vi "Set_Reset_Now.vi"(7 "I2C Channel":u8, 8 "error in (no error)":errorcluster, 11 "LINX Resource In":T1) -> (0 "error out":errorcluster, 3 "LINX Resource Out":T1)   [LabVIEW 2014, in "LMH-LINX.lvlib" / "HMC6352.lvlib"]
uses:
  <vilib>/MakerHub/LINX/Public/Sensors/Orientation/Compass/HMC6352/HMC6352.lvlib
  <vilib>/MakerHub/LINX/Private/Type Defs/LINX Ref.ctl
  <vilib>/MakerHub/LINX/Private/Type Defs/Platform.ctl
  <vilib>/MakerHub/LINX/Private/Type Defs/Interface.ctl
  <vilib>/MakerHub/LINX/Private/Device/Type Defs/LINX Device Config.ctl
  <vilib>/MakerHub/LINX/Private/Device/Type Defs/TCP Config.ctl
  <vilib>/MakerHub/LINX/Private/Device/Type Defs/Channels.ctl
  <vilib>/MakerHub/LINX/Private/Local IO/LinxI2cWrite.vi
  <vilib>/MakerHub/LINX/Public/Utilities/Check Channel.vi
  <vilib>/MakerHub/LINX/Private/Utilties/Generate Error.vi
  <vilib>/MakerHub/LINX/LMH-LINX.lvlib
  <vilib>/MakerHub/LINX/Private/Device/Device.lvlib
panel:
  # "INPUTS"
  # "OUTPUTS"
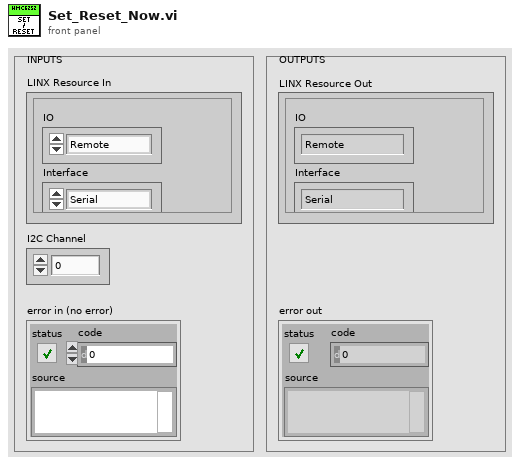
[diagram p1: front panel]
types:
  T1 = typedef "LMH-LINX.lvlib/LINX Ref.ctl" = cluster{"IO":T2, "Interface":T3, "LINX Device Config":T4}
  T2 = typedef "LMH-LINX.lvlib/Platform.ctl" = enum16{"Remote", "Local"}
  T3 = typedef "LMH-LINX.lvlib/Interface.ctl" = enum16{"Serial", "TCP"}
  T4 = typedef "LMH-LINX.lvlib/Device.lvlib/LINX Device Config.ctl" = cluster{"Interface":T3, "COM Port":refnum<visa-resource-name>, "TCP Configuration":T5, "Device Family":u8, "Device ID":u8, "Device Name":string, "TCP Ref":refnum<k5>, "Channels":T6}
  T5 = typedef "LMH-LINX.lvlib/Device.lvlib/TCP Config.ctl" = cluster{"IP Address":string, "Port":u16}
  T6 = typedef "LMH-LINX.lvlib/Channels.ctl" = cluster{"DI":u8[], "DO":u8[], "AI":u8[], "AO":u8[], "PWM":u8[], "QE":u8[], "UART":u8[], "I2C 2":u8[], "SPI":u8[], "CAN":u8[], "Servo":u8[], "AI Ref (V)":dbl, "AI Resolution (Bits)":u8, "AO Ref (V)":dbl, "AO Resolution (Bits)":u8}
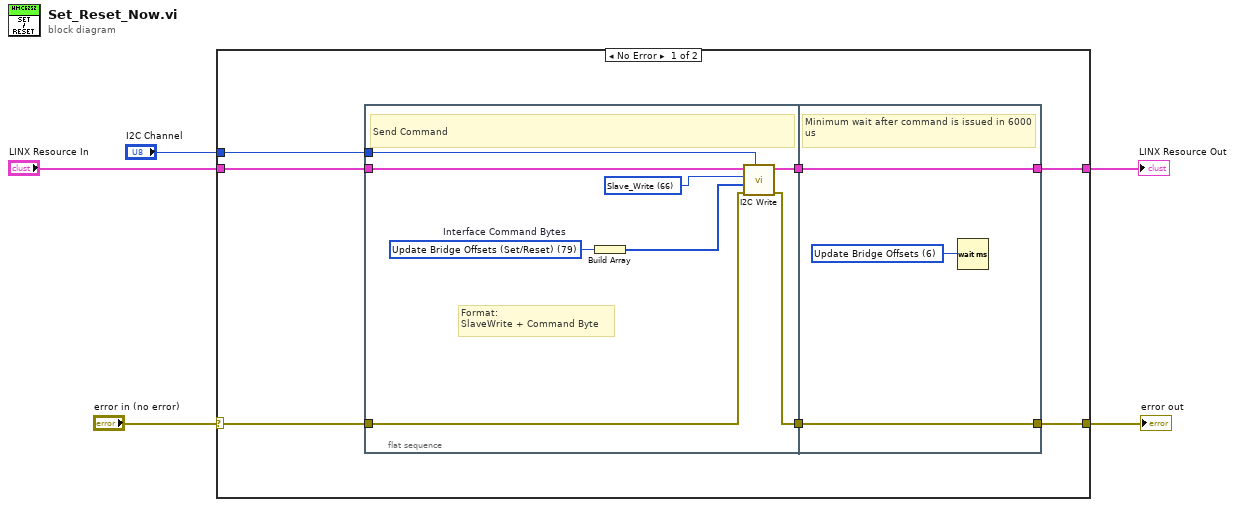
[diagram p0: block diagram]
diagram:
  n1 = case shown="No Error" "error in (no error)" {
    selector: "error in (no error)" -> [w10 w25]
    tunnel: [w8 w25] -> w4
    tunnel: "LINX Resource In" -> [w12 w24]
    tunnel: "I2C Channel" -> [w11 _]
    tunnel: [w9 w24] -> w1
    frame No Error {
      n2 = flat-sequence {
        tunnel: w12 -> [w20]
        tunnel: w11 -> [w19]
        tunnel: w10 -> [w18]
        tunnel: [w17] -> w7
        tunnel: [w16] -> w6
        tunnel: [w22] -> w8
        tunnel: [w23] -> w9
        tunnel: w7 -> [w23]
        tunnel: w6 -> [w22]
        frame #0 {
          w14 = u8 79 items=["Write to EEPROM"=119, "Read from EEPROM"=114, "Write to RAM Register"=71, "Read from RAM Register"=103, "Enter Sleep Mode"=83, "Exit Sleep Mode"=87, "Update Bridge Offsets (Set/Reset)"=79, "Enter User Calibration Mode"=67, "Exit User Calibration Mode"=69, "Save Operation Mode to EEPROM"=76, "J_Who_am_i"=117, "Get Data/Calculate New Heading"=65]  # Interface Command Bytes
          w13 = u8 66 items=["Slave_Write"=66, "Slave_Read"=67] ("HMC6352 Slave Address")
          # "Format:\nSlaveWrite + Command Byte"
          # "Send Command"
          n3 = Build Array(w14) -> (w15:u8[])
          n4 = call <vilib>:"I2C Write.vi"("I2C Channel"=w19, "Error In"=w18, "Data"=w15, "I2C Slave Address (0)"=w13, "LINX Resource"=w20) -> ("Error Out"=w16:errorcluster, "LINX Resource"=w17:T1)  [unwired: 5 in]
        }
        frame #1 {
          w21 = u32 6 items=["Update Bridge Offsets"=6, "Exit User Calibration Mode"=14, "Get New Heading"=0] ("Command Time Delays (ms)")
          # "Minimum wait after command is issued in 6000 us"
          n5 = Wait (ms)(milliseconds to wait=w21) -> ()  [unwired: 1 out]
        }
      }
    }
    frame Error {
    }
  }
  "error out" <- w4
  "LINX Resource Out" <- w1
